vi "NF WF1973_74 OUTP.vi"(6 "Read(F)":bool, 8 "error in (no error)":errorcluster caption="Error IN", 9 "Output(OFF)":bool, 10 "Ch(Ch1)":bool, 11 "VISAsession":refnum<visa-resource-name>) -> (0 "error out":errorcluster caption="Error OUT", 2 "Query State":i32=9, 3 "CopyVISAsession":refnum<visa-resource-name>)   [LabVIEW 2010]
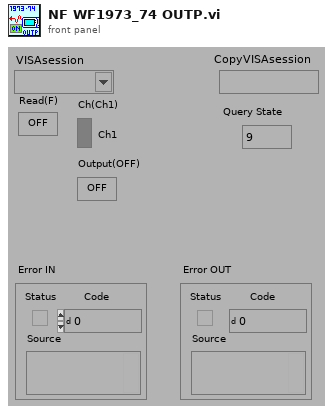
[diagram p1: front panel]
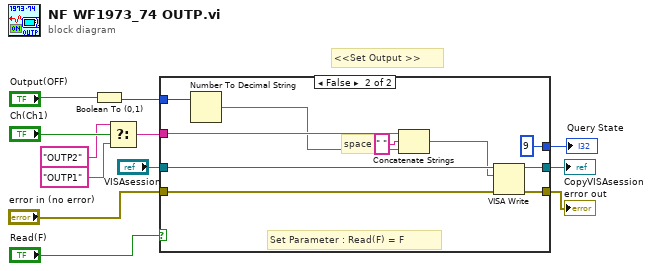
[diagram p0: block diagram]
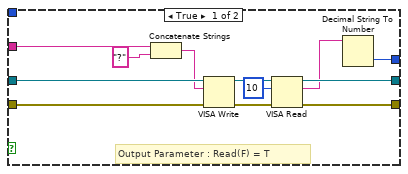
[diagram p2: hidden frame]
diagram:
  # "<<Set Output >>"
  n1 = Boolean To (0,1)(Boolean="Output(OFF)") -> (0, 1=w1:i16)
  n2 = Select(t="OUTP2" ("文字列"), s="Ch(Ch1)", f="OUTP1" ("文字列")) -> (s? t:f=w5:string)
  n3 = case shown="FALSE" "Read(F)" {
    tunnel: "VISAsession" -> [w24 w34]
    tunnel: [w21 w32] -> w11
    tunnel: [w20 w33] -> w10
    tunnel: "error in (no error)" -> [w19 w31]
    tunnel: w5 -> [w17 w27]
    tunnel: [w14 9] -> w7
    tunnel: w1 -> [_ w29]
    frame True {
      # "Output Parameter : Read(F) = T"
      n4 = Concatenate Strings(w17, "?" ("形式文字列")) -> (w15:string)
      n5 = VISA Write(VISA resource name=w24, write buffer=w15, error in (no error)=w19) -> (VISA resource name out=w22:refnum<visa-resource-name>, error out=w23:errorcluster)  [unwired: 1 out]
      n6 = VISA Read(VISA resource name=w22, byte count=u32 10 ("バイトカウント（0）"), error in (no error)=w23) -> (VISA resource name out=w21:refnum<visa-resource-name>, read buffer=w13:string, error out=w20:errorcluster)  [unwired: 1 out]
      n7 = Decimal String To Number(string=w13) -> (number=w14:i32)  [unwired: 2 in, 1 out]
    }
    frame False {
      # "space"
      # "Set Parameter : Read(F) = F"
      n8 = Number To Decimal String(number=w29) -> (decimal integer string=w25:string)  [unwired: 1 in]
      n9 = Concatenate Strings(w27, " " ("文字列"), w25) -> (w28:string)
      n10 = VISA Write(VISA resource name=w34, write buffer=w28, error in (no error)=w31) -> (VISA resource name out=w32:refnum<visa-resource-name>, error out=w33:errorcluster)  [unwired: 1 out]
    }
  }
  "error out" <- w10
  "CopyVISAsession" <- w11
  "Query State" <- w7
